vi "Close VI FP.vi"(8 "error in (no error)":errorcluster, 11 "path":path) -> (0 "error out":errorcluster)   [LabVIEW 2014, in "Raspberry Pi Compatible Compiler for LabVIEW.lvlib"]
uses:
  Raspberry Pi Compatible Compiler for LabVIEW.lvlib
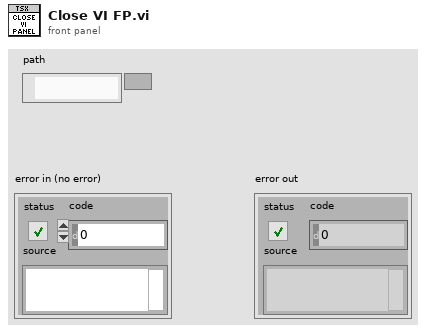
[diagram p1: front panel]
types:
  T1 = enum32{"Invalid", "Standard", "Closed", "Hidden", "Minimized", "Maximized"}
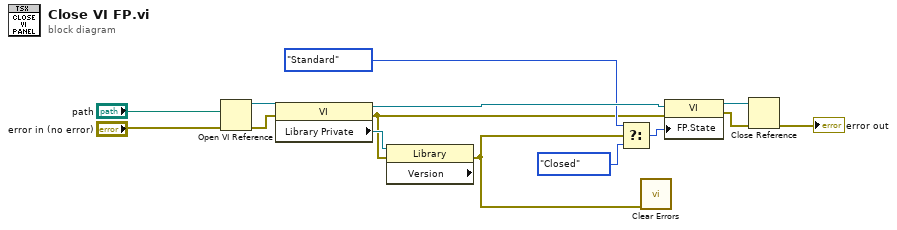
[diagram p0: block diagram]
diagram:
  n1 = Open VI Reference(vi path="path", error in (no error)="error in (no error)") -> (vi reference=w9:refnum<vi>, error out=w8:errorcluster)  [unwired: 4 in]
  n2 = property class="VI"(reference=w9, error in=w8) -> (reference out=w7:refnum<vi>, error out=w2:errorcluster, "Library Private"=w3:refnum<vi>)
  n3 = property class="Library" props=["Version"](reference=w3, error in=w2) -> (error out=w1:errorcluster)  [unwired: 2 out]
  n4 = Select(t=T1."Standard" ("Front Panel Window:State"), s=w1, f=T1."Closed" ("Front Panel Window:State")) -> (s? t:f=w4:T1)
  n5 = call <vilib>:"Clear Errors.vi"("error in (no error)"=w1) -> ()  [unwired: 5 in, 2 out]
  n6 = property class="VI"(reference=w7, error in=w2, "FP.State"=w4) -> (reference out=w11:refnum<vi>, error out=w12:errorcluster)
  n7 = Close Reference(reference=w11, error in (no error)=w12) -> (error out=→"error out":errorcluster)
